vi "CorrectResponse.vi"(8 "error in (no error)":errorcluster, 11 "TrialBasedExperiment in":refnum<class "ClassDiscrimination.lvclass">) -> (0 "error out":errorcluster, 3 "TrialBasedExperiment out":refnum<class "ClassDiscrimination.lvclass">)   [LabVIEW 2011, in "ClassDiscrimination.lvclass"]
uses:
  ClassDiscrimination.lvclass
  Trial Based Experiment Statechart/MatlabExperiment/MatlabExperiment.lvclass
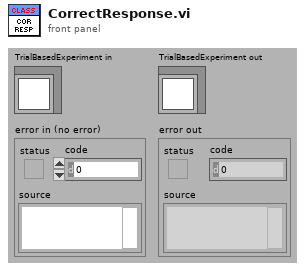
[diagram p1: front panel]
types:
  T1 = cluster{"Intertrial":dbl, "AcquireFixation":dbl, "HoldFixation":dbl, "DelayPeriod":dbl, "ResponsePeriod":dbl}
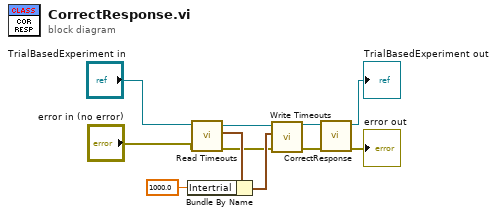
[diagram p0: block diagram]
diagram:
  n1 = call-dynamic "Read Timeouts.vi"("error in (no error)"="error in (no error)", "TrialBasedExperiment in"="TrialBasedExperiment in") -> ("error out"=w5:errorcluster, "Timeouts"=w9:T1, "TrialBasedExperiment out"=w6:refnum<class "ClassDiscrimination.lvclass">)  [unwired: 7 in]
  n2 = Bundle By Name(cluster=w9, "Intertrial"=1000.0) -> (w7:T1)
  n3 = call-dynamic "Write Timeouts.vi"("error in (no error)"=w5, "Timeouts"=w7, "TrialBasedExperiment in"=w6) -> ("error out"=w3:errorcluster, "TrialBasedExperiment out"=w4:refnum<class "ClassDiscrimination.lvclass">)  [unwired: 7 in]
  n4 = call-parent "CorrectResponse.vi"("error in (no error)"=w3, "TrialBasedExperiment in"=w4) -> ("error out"=→"error out":errorcluster, "TrialBasedExperiment out"=→"TrialBasedExperiment out":refnum<class "ClassDiscrimination.lvclass">)  [unwired: 8 in]
